vi "Sect02-Single File_Write ROI Image and Overlay.vi"(8 "error in (no error)":errorcluster, 9 "ROI Descriptor":T1 {"Contours"."Type" items=["No Selection", "Point", "Line", "Rectangle", "Oval", "Polygon", "Freehand Region", "Annulus", "Unused2", "Unused3", "Broken Line", "Freehand Line", "Rotated Rectangle"]}, 10 "ROI Image (with overlay)":T2, 11 "QSM_ShiftRegister_TEST in":T3 {"ROI Process"."Particle Variables" items=["Center of Mass X", "Center of Mass Y", "First Pixel X", "First Pixel Y", "Bounding Rect Left", "Bounding Rect Top", "Bounding Rect Right", "Bounding Rect Bottom", "Max Feret Diameter Start X", "Max Feret Diameter Start Y", "Max Feret Diameter End X", "Max Feret Diameter End Y", "Max Horiz. Segment Length Left", "Max Horiz. Segment Length Right", "Max Horiz. Segment Length Row", "-", "Bounding Rect Width", "Bounding Rect Height", "Bounding Rect Diagonal", "Perimeter", "Convex Hull Perimeter", "Holes' Perimeter", "Max Feret Diameter", "Equivalent Ellipse Major Axis", "Equivalent Ellipse Minor Axis", "Equivalent Ellipse Minor Axis (Feret)", "Equivalent Rect Long Side", "Equivalent Rect Short Side", "Equivalent Rect Diagonal", "Equivalent Rect Short Side (Feret)", "Average Horiz. Segment Length", "Average Vert. Segment Length", "Hydraulic Radius", "Waddel Disk Diameter", "-", "Area", "Holes' Area", "Particle & Holes' Area", "Convex Hull Area", "Image Area", "-", "Number of Holes", "Number of Horiz. Segments", "Number of Vert. Segments", "-", "Orientation", "Max Feret Diameter Orientation", "-", "% Area/Image Area", "% Area/(Particle & Holes' Area)", "Ratio of Equivalent Ellipse Axes", "Ratio of Equivalent Rect Sides", "-", "Elongation Factor", "Compactness Factor", "Heywood Circularity Factor", "Type Factor", "-", "Sum X", "Sum Y", "Sum XX", "Sum XY", "Sum YY", "Sum XXX", "Sum XXY", "Sum XYY", "Sum YYY", "-", "Moment of Inertia XX", "Moment of Inertia XY", "Moment of Inertia YY", "Moment of Inertia XXX", "Moment of Inertia XXY", "Moment of Inertia XYY", "Moment of Inertia YYY", "Norm. Moment of Inertia XX", "Norm. Moment of Inertia XY", "Norm. Moment of Inertia YY", "Norm. Moment of Inertia XXX", "Norm. Moment of Inertia XXY", "Norm. Moment of Inertia XYY", "Norm. Moment of Inertia YYY", "Hu Moment 1", "Hu Moment 2", "Hu Moment 3", "Hu Moment 4", "Hu Moment 5", "Hu Moment 6", "Hu Moment 7"]; "ROI Process"."Particle Measurements (Pixels)" format="%.2f"; "ROI Process"."ROIS"."Contours"."Type" items=["No Selection", "Point", "Line", "Rectangle", "Oval", "Polygon", "Freehand Region", "Annulus", "Unused2", "Unused3", "Broken Line", "Freehand Line", "Rotated Rectangle"]; "Single Image Results"."ROI Results"."LIMLOCALMETADATA"."dTimeMSec" format="%.2f"}) -> (0 "error out":errorcluster, 3 "QSM_ShiftRegister_TEST out":T3 {"ROI Process"."Particle Variables" items=["Center of Mass X", "Center of Mass Y", "First Pixel X", "First Pixel Y", "Bounding Rect Left", "Bounding Rect Top", "Bounding Rect Right", "Bounding Rect Bottom", "Max Feret Diameter Start X", "Max Feret Diameter Start Y", "Max Feret Diameter End X", "Max Feret Diameter End Y", "Max Horiz. Segment Length Left", "Max Horiz. Segment Length Right", "Max Horiz. Segment Length Row", "-", "Bounding Rect Width", "Bounding Rect Height", "Bounding Rect Diagonal", "Perimeter", "Convex Hull Perimeter", "Holes' Perimeter", "Max Feret Diameter", "Equivalent Ellipse Major Axis", "Equivalent Ellipse Minor Axis", "Equivalent Ellipse Minor Axis (Feret)", "Equivalent Rect Long Side", "Equivalent Rect Short Side", "Equivalent Rect Diagonal", "Equivalent Rect Short Side (Feret)", "Average Horiz. Segment Length", "Average Vert. Segment Length", "Hydraulic Radius", "Waddel Disk Diameter", "-", "Area", "Holes' Area", "Particle & Holes' Area", "Convex Hull Area", "Image Area", "-", "Number of Holes", "Number of Horiz. Segments", "Number of Vert. Segments", "-", "Orientation", "Max Feret Diameter Orientation", "-", "% Area/Image Area", "% Area/(Particle & Holes' Area)", "Ratio of Equivalent Ellipse Axes", "Ratio of Equivalent Rect Sides", "-", "Elongation Factor", "Compactness Factor", "Heywood Circularity Factor", "Type Factor", "-", "Sum X", "Sum Y", "Sum XX", "Sum XY", "Sum YY", "Sum XXX", "Sum XXY", "Sum XYY", "Sum YYY", "-", "Moment of Inertia XX", "Moment of Inertia XY", "Moment of Inertia YY", "Moment of Inertia XXX", "Moment of Inertia XXY", "Moment of Inertia XYY", "Moment of Inertia YYY", "Norm. Moment of Inertia XX", "Norm. Moment of Inertia XY", "Norm. Moment of Inertia YY", "Norm. Moment of Inertia XXX", "Norm. Moment of Inertia XXY", "Norm. Moment of Inertia XYY", "Norm. Moment of Inertia YYY", "Hu Moment 1", "Hu Moment 2", "Hu Moment 3", "Hu Moment 4", "Hu Moment 5", "Hu Moment 6", "Hu Moment 7"]; "ROI Process"."Particle Measurements (Pixels)" format="%.2f"; "ROI Process"."ROIS"."Contours"."Type" items=["No Selection", "Point", "Line", "Rectangle", "Oval", "Polygon", "Freehand Region", "Annulus", "Unused2", "Unused3", "Broken Line", "Freehand Line", "Rotated Rectangle"]; "Single Image Results"."ROI Results"."LIMLOCALMETADATA"."dTimeMSec" format="%.2f"})   [LabVIEW 2014, in "TestQSM.lvlib"]
uses:
  TestQSM.lvlib
  Controls/QSM_ShiftRegister.ctl
  QueueMaintenance/TypeDef/QSMRef_ALL.ctl
  Queue_TESTGUIUPDATE/Controls/QSM_Reference.ctl
  Queue_TESTGUIUPDATE/Controls/QSM_DataType.ctl
  Queue_TESTGUIUPDATE/Controls/QSM_RunStates.ctl
  Controls/QSM_Reference.ctl
  Controls/QSM_DataType.ctl
  Controls/QSM_RunStates.ctl
  Custom Controls/cluster - Image Results.ctl
  ND2_Reader_32bit/controls/cluster_LIMLOCALMETADATA.ctl
  <vilib>/vision/Image Controls.llb/IMAQ Image.ctl
  FileIO/TypeDef - File Actions.ctl
  Queue_TESTGUIUPDATE/GUIUpdateQSM.lvlib
  QueueMaintenance/QueueMaintenance.lvlib
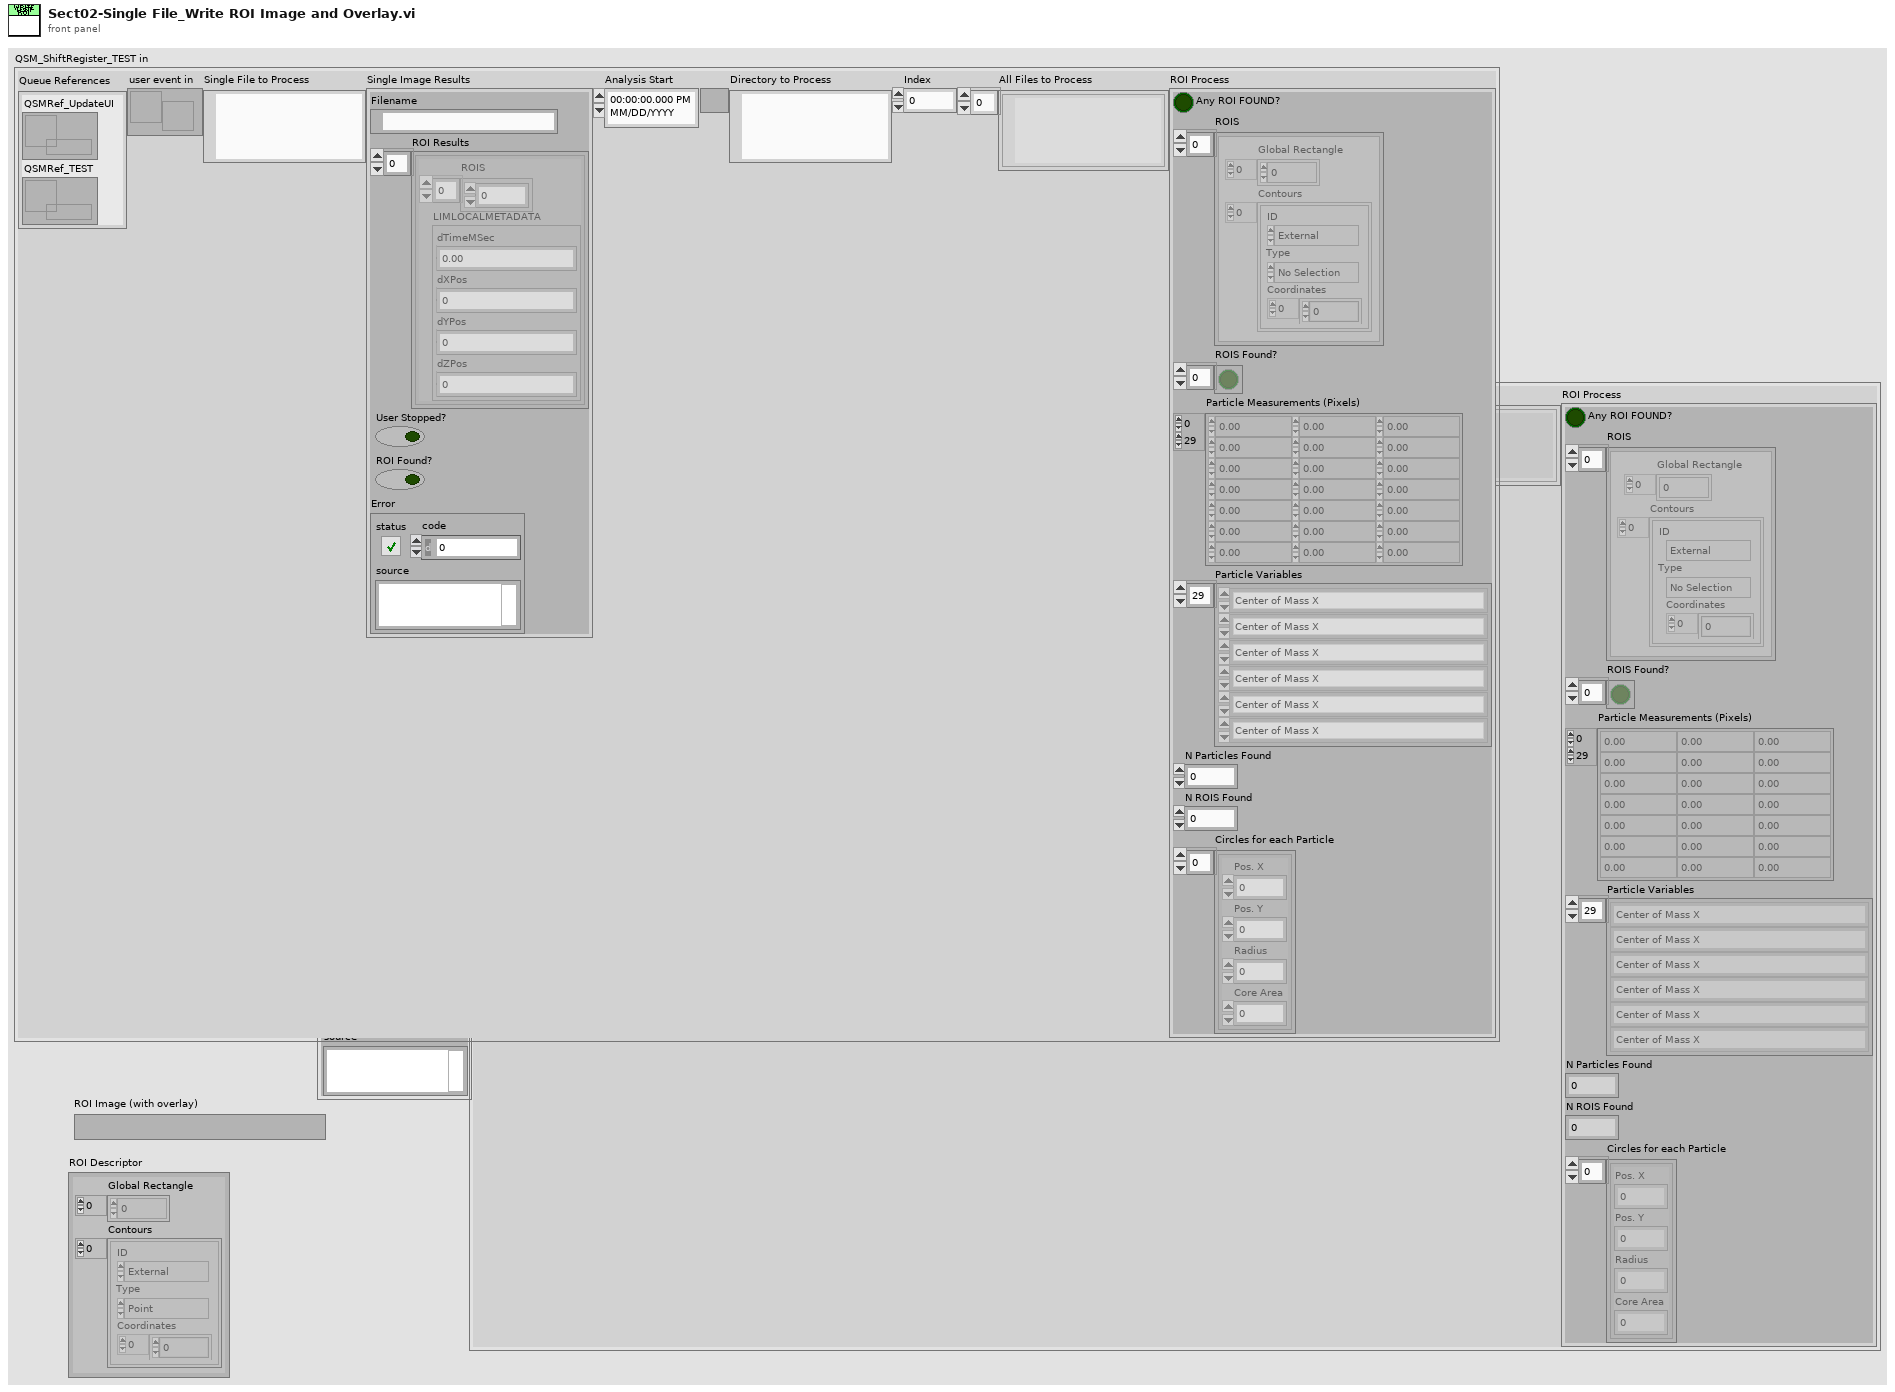
[diagram p1: front panel]
types:
  T1 = typedef "ROI Descriptor" = cluster{"Global Rectangle":i32[], "Contours":cluster{"ID":enum32{"External", "Internal"}, "Type":u32, "Coordinates":i32[]}[]}
  T2 = typedef "IMAQ Image.ctl" = refnum<image>
  T3 = typedef "TestQSM.lvlib/QSM_ShiftRegister.ctl" = cluster{"Queue References":T4, "user event in":refnum<user-event>, "Single File to Process":path, "Single Image Results":T7, "Analysis Start":timestamp, "Directory to Process":path, "Index":i32, "All Files to Process":path[], "ROI Process":cluster{"Any ROI FOUND?":bool, "ROIS":T1[], "ROIS Found?":bool[], "Particle Measurements (Pixels)":dbl[][], "Particle Variables":i32[], "N Particles Found":i32, "N ROIS Found":i32, "Circles for each Particle":cluster{"Pos. X":i32, "Pos. Y":i32, "Radius":i32, "Core Area":i32}[]}}
  T4 = typedef "QueueMaintenance.lvlib/QSMRef_ALL.ctl" = cluster{"QSMRef_UpdateUI":T5, "QSMRef_TEST":T6}
  T5 = typedef "GUIUpdateQSM.lvlib/QSM_Reference.ctl" = refnum<queue>
  T6 = typedef "TestQSM.lvlib/QSM_Reference.ctl" = refnum<queue>
  T7 = typedef "cluster - Image Results.ctl" = cluster{"Filename":path, "ROI Results":cluster{"ROIS":dbl[], "LIMLOCALMETADATA":T8}[], "User Stopped?":bool, "ROI Found?":bool, "Error":errorcluster}
  T8 = typedef "cluster_LIMLOCALMETADATA.ctl" = cluster{"dTimeMSec":dbl, "dXPos":dbl, "dYPos":dbl, "dZPos":dbl}
  T9 = enum32{"Gray", "Binary", "Gradient", "Rainbow", "Temperature"}
  T10 = typedef "Image Type" = u32
  T11 = typedef "TypeDef - File Actions.ctl" = enum16{"Read", "Write", "Get Current"}
  T12 = typedef "TypeDef - System Configuration.ctl" = cluster{"Results FilePath":path, "Analysis Parameters":cluster{"Area":cluster{"Lower Value":dbl, "Upper Value":dbl}, "Circle Filter Radius":cluster{"Lower Value":sgl, "Upper Value":sgl}, "Edge Detection Threshold":u16}, "ROI Parameters":cluster{"ROI size (in Radius)":cluster{"Width":dbl, "Height":dbl}}}
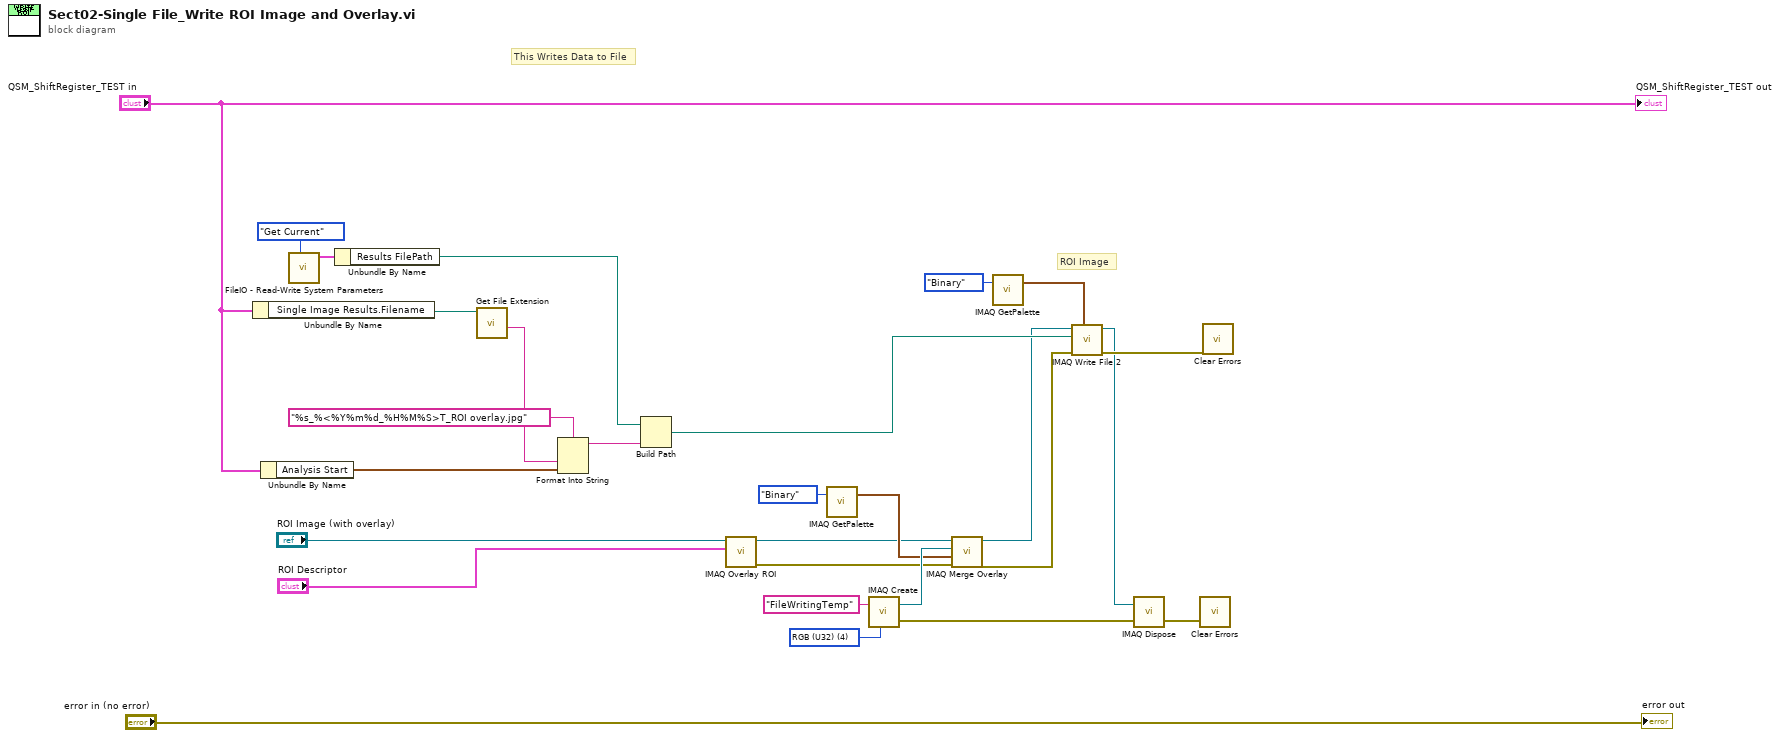
[diagram p0: block diagram]
diagram:
  w13 = T10 4 items=["Grayscale (U8)", "Grayscale (I16)", "Grayscale (SGL)", "Complex (CSG)", "RGB (U32)", "HSL (U32)", "RGB (U64)", "Grayscale (U16)"] ("Image Type")
  # "ROI Image"
  # "This Writes Data to File"
  n1 = Unbundle By Name("QSM_ShiftRegister_TEST in") -> ("Single Image Results.Filename"=w27:path)
  n2 = Unbundle By Name("QSM_ShiftRegister_TEST in") -> ("Analysis Start"=w20:timestamp)
  n3 = call "FileIO - Read-Write System Parameters.vi"("Action"=TypeDef_-_File_Actions."Get Current") -> ("System Parameters out"=w25:T12)  [unwired: 9 in, 1 out]
  n4 = Unbundle By Name(w25) -> ("Results FilePath"=w19:path)
  n5 = call <vilib>:"Get File Extension.vi"("file"=w27) -> ("filename without extension"=w21:string)  [unwired: 7 in, 3 out]
  n6 = Format Into String(format string="%s_%<%Y%m%d_%H%M%S>T_ROI overlay.jpg", w21, w20) -> (resulting string=w23:string)  [unwired: 2 in, 1 out]
  n7 = Build Path(base path=w19, name or relative path=w23) -> (appended path=w18:path)
  n8 = call "IMAQ Overlay ROI"("ROI Descriptor"="ROI Descriptor", "Image"="ROI Image (with overlay)") -> ("error out"=w2:errorcluster, "Image Out"=w5:T2)  [unwired: 8 in]
  n9 = call "IMAQ GetPalette"("Palette Number (gray)"=T9."Binary") -> ("Color Palette"=w9:cluster{"Red":u8, "Green":u8, "Blue":u8}[])  [unwired: 4 in, 1 out]
  n10 = call "IMAQ Create"("Image Name"="FileWritingTemp", "Image Type"=w13) -> ("New Image"=w14:T2, "error out"=w12:errorcluster)  [unwired: 3 in]
  n11 = call "IMAQ Merge Overlay"("error in (no error)"=w2, "Color Palette"=w9, "Image Dst"=w14, "Image Src"=w5) -> ("error out"=w1:errorcluster, "Image Dst Out"=w8:T2)  [unwired: 6 in]
  n12 = call "IMAQ GetPalette"("Palette Number (gray)"=T9."Binary") -> ("Color Palette"=w15:cluster{"Red":u8, "Green":u8, "Blue":u8}[])  [unwired: 4 in, 1 out]
  n13 = call-poly "IMAQ Write File 2"("Color Palette"=w15, "error in (no error)"=w1, "File Path"=w18, "Image"=w8) -> ("error out"=w17:errorcluster, "Image Out (duplicate)"=w7:T2)  [unwired: 6 in]
  n14 = call "IMAQ Dispose"("Image"=w7, "error in (no error)"=w12) -> ("error out"=w3:errorcluster)  [unwired: 4 in]
  n15 = call <vilib>:"Clear Errors.vi"("error in (no error)"=w3) -> ()  [unwired: 5 in, 2 out]
  n16 = call <vilib>:"Clear Errors.vi"("error in (no error)"=w17) -> ()  [unwired: 5 in, 2 out]
  "error out" <- "error in (no error)"
  "QSM_ShiftRegister_TEST out" <- "QSM_ShiftRegister_TEST in"
